vi "LVDT Thickness.vi"() -> ()   [LabVIEW 2014]
uses:
  <vilib>/Utility/miscctls.llb/LVBoundsTypeDef.ctl
  <vilib>/measure/NI_MABase.lvlib
panel:
  in  "stop":bool
  out "x >= y?":bool
  in  "Tab Control":T1(tab)
  out "Stage 2 Output":dbl(graph)
  out "Stage 1 Output":waveform(dbl)(graph)
  in  "?":bool
  in  "Slide":dbl(slide)=0.14061224489795918 scale=0.0..13.78
  out "?":dbl(slide) scale=0.0..15.0
  out "?":dbl format="%#_4g"
  out "?":dbl format="%#_4g"
  out "?":bool
  in  "?":bool
  out "?":dbl format="%#_4g"
  in  "?":dbl(slide)=29.292929292929294 scale=0.0..100.0
  out "?":dbl(slide) scale=0.0..15.0
  out "?":dbl format="%#_4g"
  out "Thickness (in mm) Vs Voltage (V)":cluster{"Y":dbl[], "Y":dbl[]}[](graph)
  out "1 2":string[][](table)
  out "?":bool
  out "Stage 1 Output  2":waveform(dbl)(graph)
  out "Stage 2 Output  2":dbl(graph)
  # "Manipal Institute of Technology  \n        Dept of Instrumentation and Control Engineering\n                                 V Sem (Instrumentation Lab)"
  # "VIRTUAL LABS"
  # "VIRTUAL LABS"
  # "Measurement of Level Using Ultrasonic Transducer\n \nAim:\nTo measure the liquid level in the process tank using Ultrasonic Transducer.\n Apparatus required:\n1\tVLMT-04 Unit.\n2\tPatch Chord.\n3\tDMM\n\n\nInstructions:\n1.\tSwitch ON the Trainer. \n2.\tThe Pump inlet valve (HV1) should be fully open and the process tank outlet valve HV2 should be fully closed. \n3.\tConnect the multimeter across (4-20) mA.\n4.\tVary the pump speed using variable speed knob, set the level at 0mm. \n5.\tNote the transmitter output in (4-20) mA terminals.\n6.\tGradually increase the water level by using variable speed knob and note down the water level and transmitter output.\n7.\tPlot the Graph between level (mm) and transmitter output (mA) along x-axis and y-axis respectively."
  # "EXPERIMENT NO.1"
  # "Thickness (mm)"
  # "Voltage o/p (V)"
  # "Thickness (mm)"
  # "Voltage o/p (V)"
  # "Animation Speed"
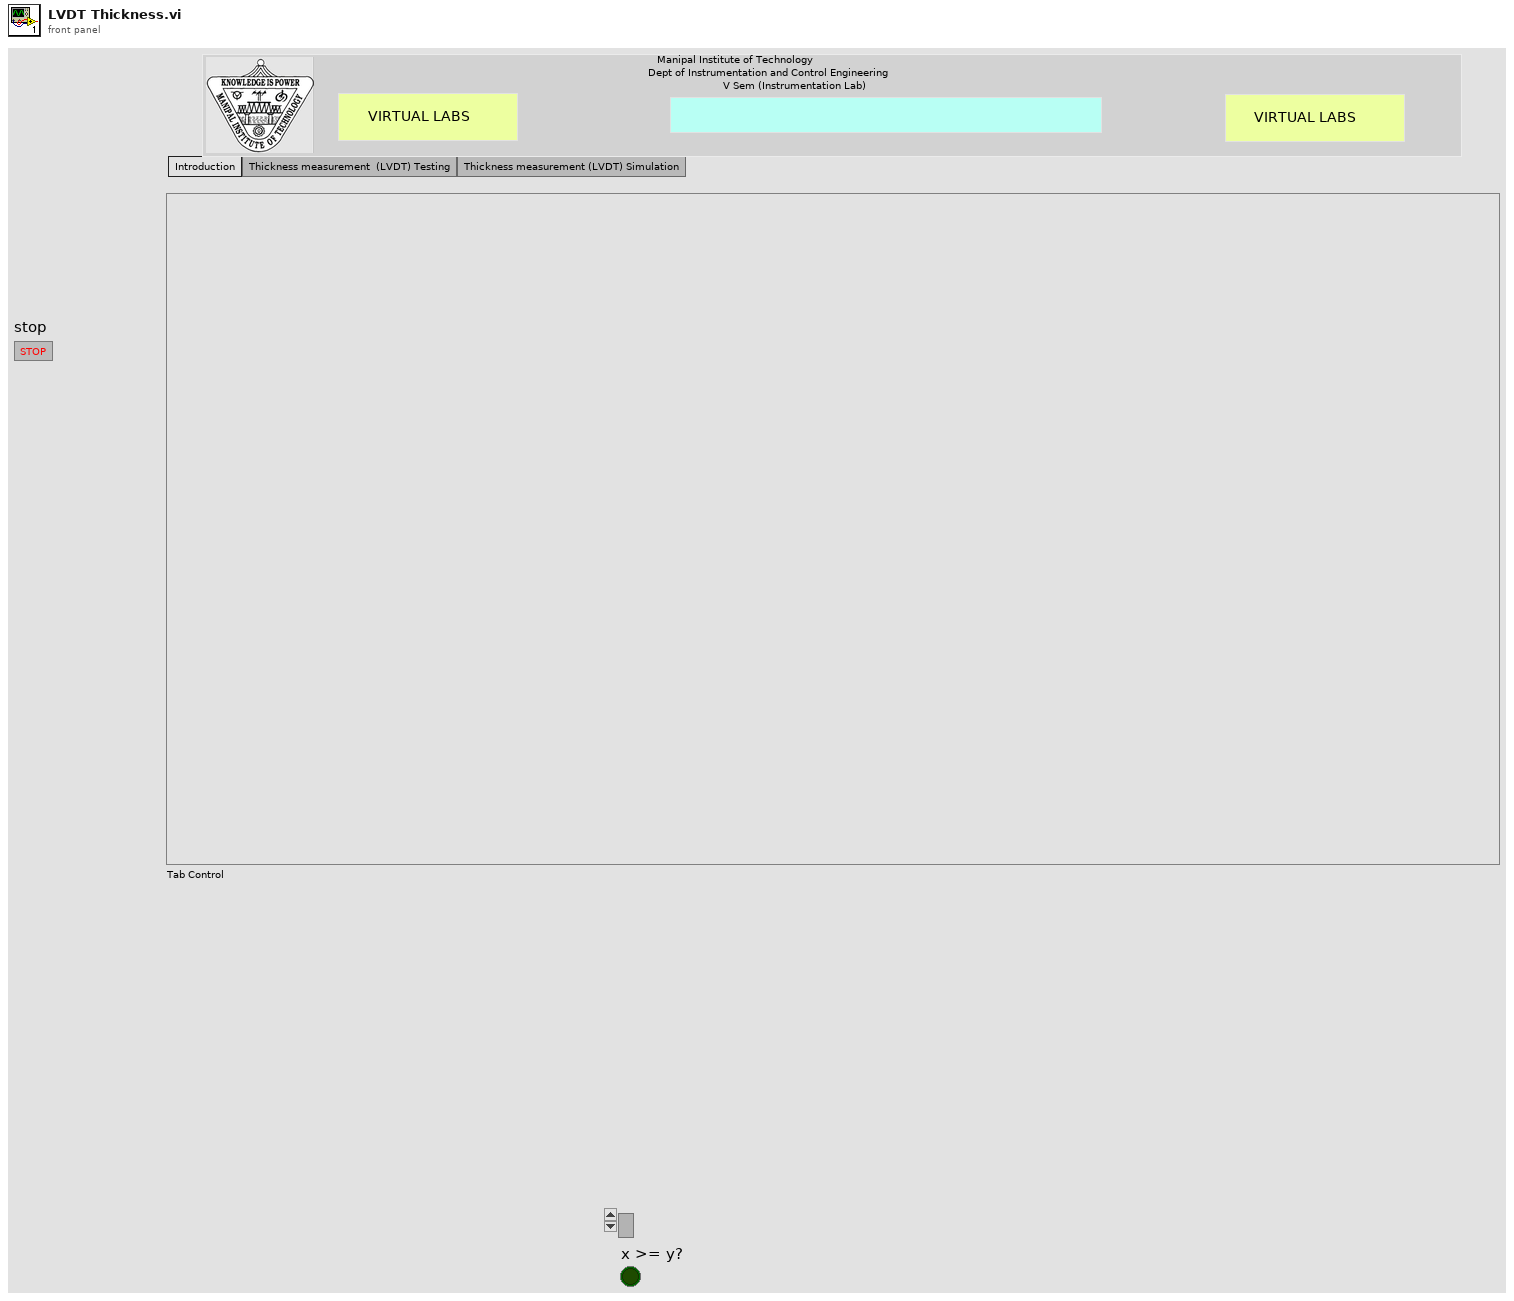
[diagram p1: front panel]
types:
  T1 = enum32{"Introduction", "Thickness measurement  (LVDT) Testing", "Thickness measurement (LVDT) Simulation"}
  T2 = typedef "LVBoundsTypeDef.ctl" = cluster{"Width":u32, "Height":u32}
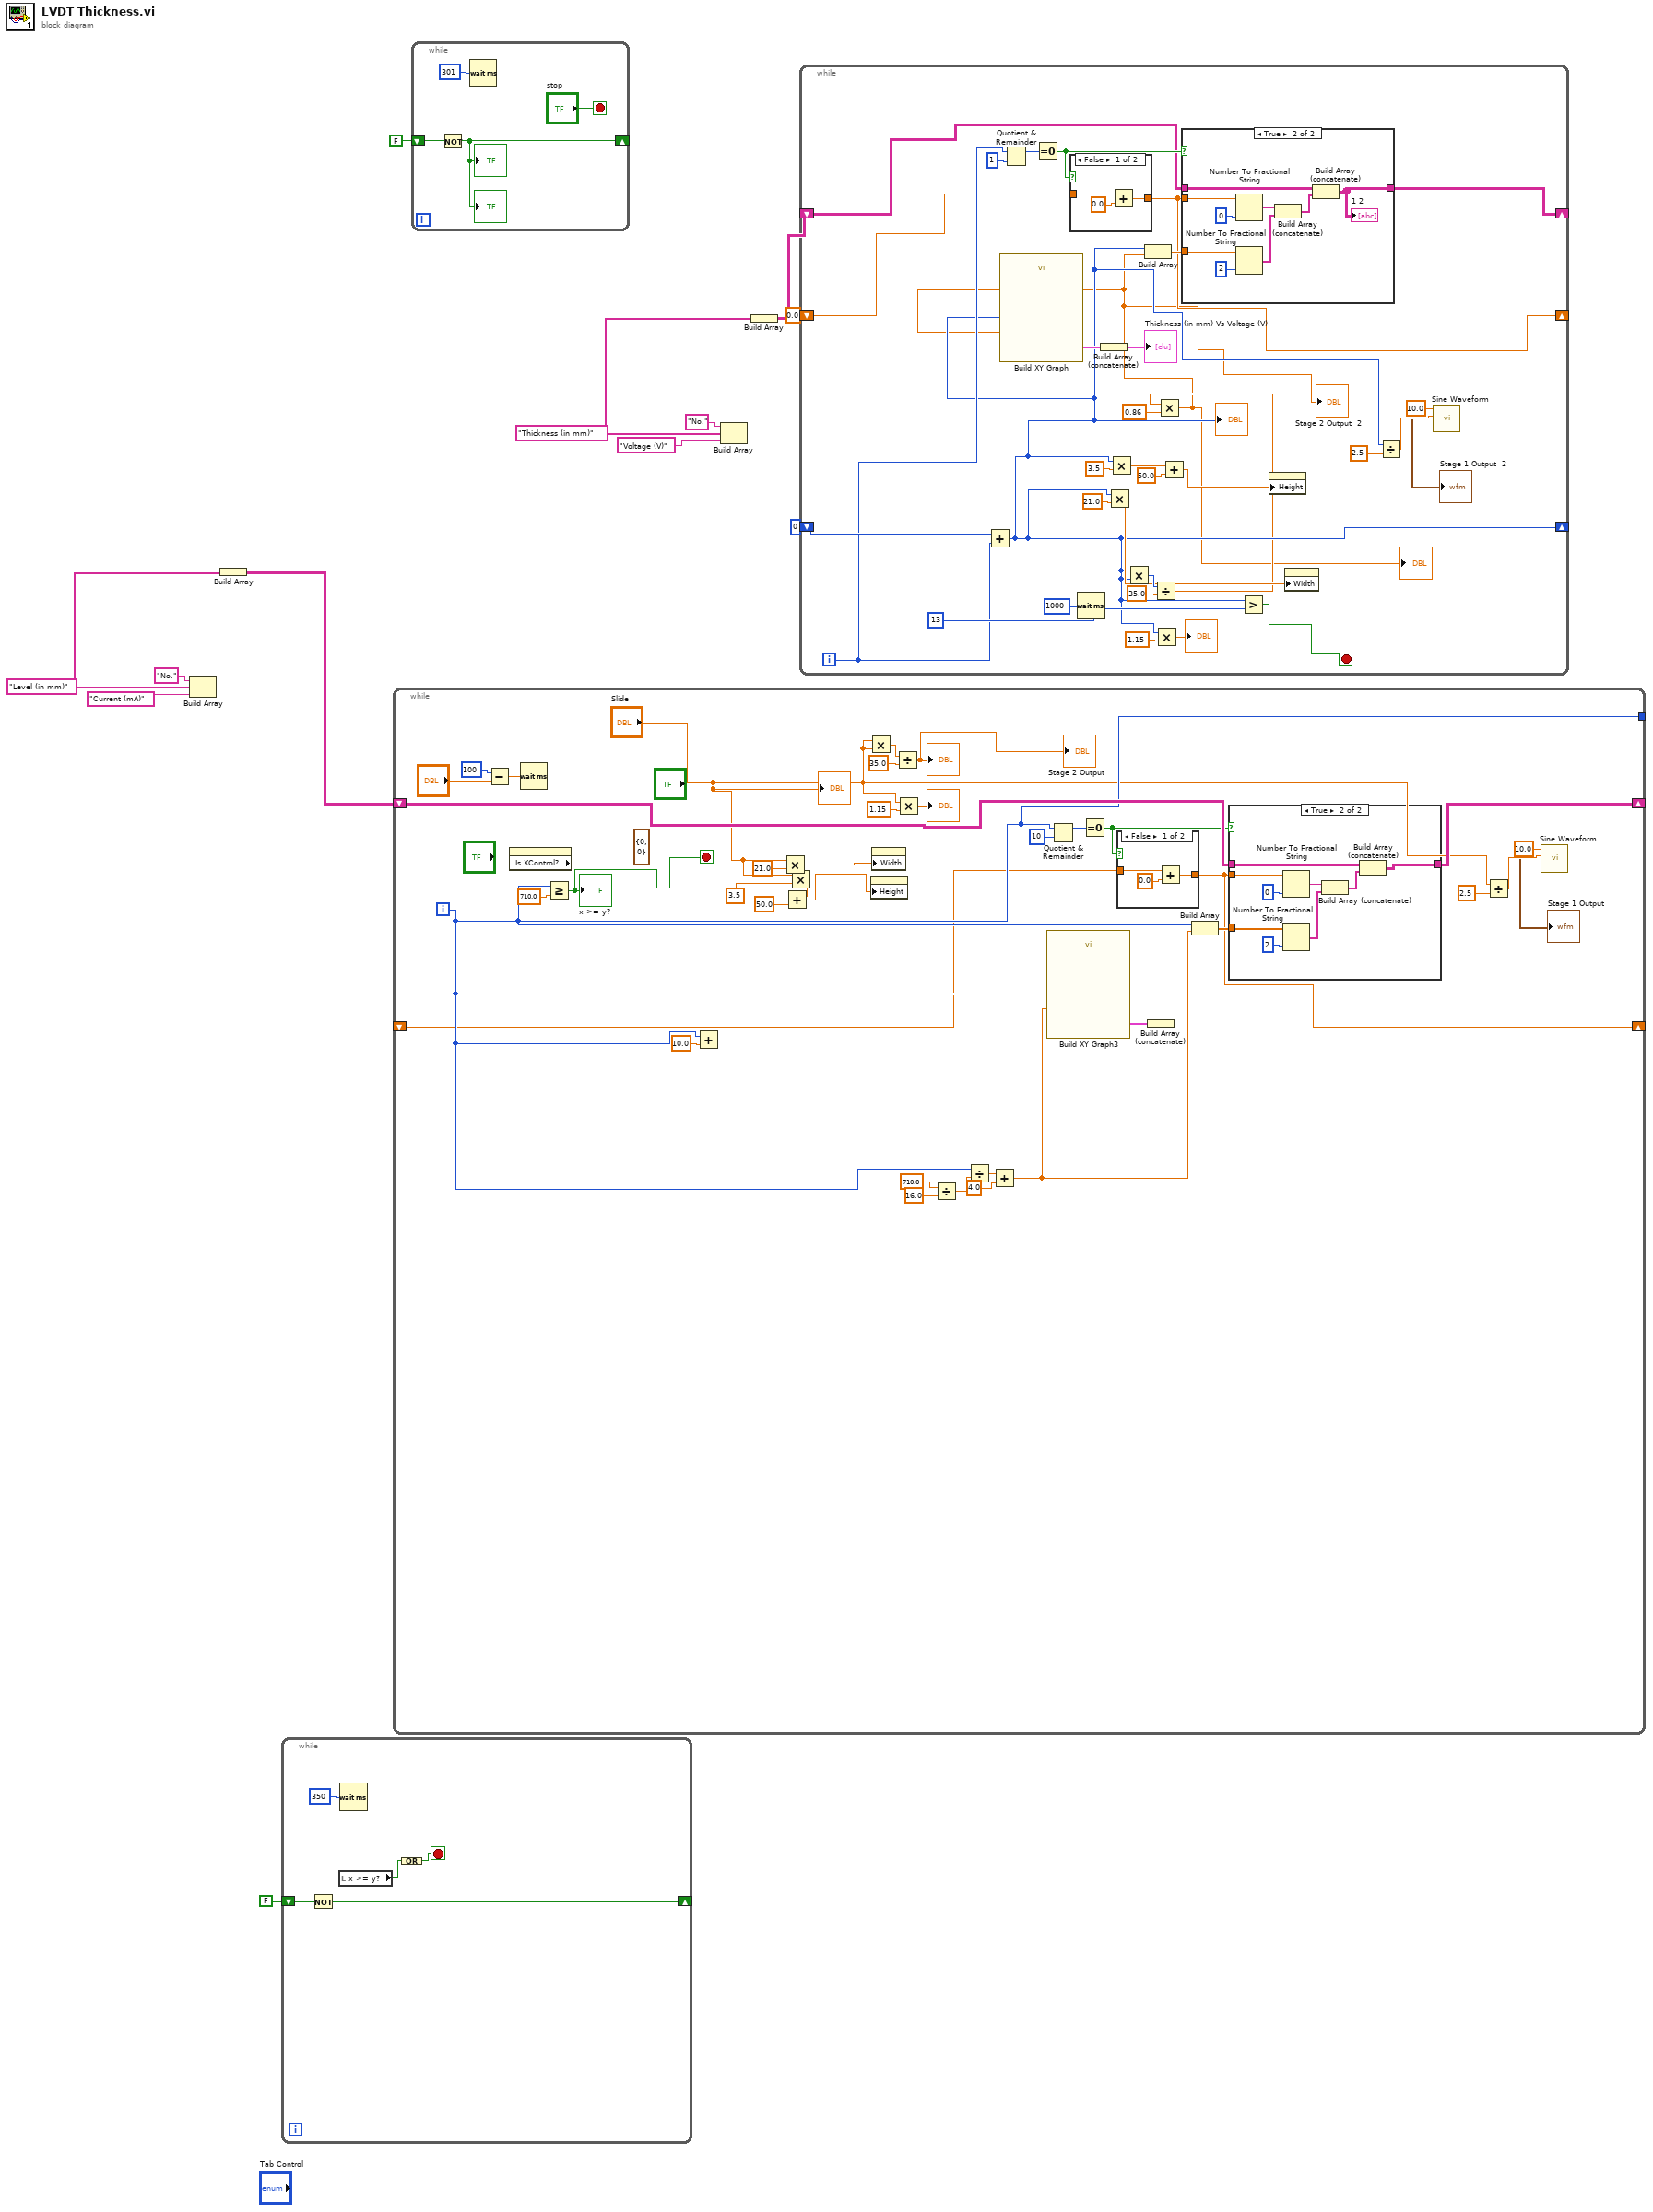
[diagram p0: block diagram]
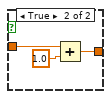
[diagram p2: hidden frame]
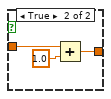
[diagram p4: hidden frame]
diagram:
  n1 = Build Array("No." ("element"), "Level (in mm)" ("element"), "Current (mA)") -> (w11:string[])
  n2 = Build Array(w11) -> (w10:string[][])
  n3 = while {
    shift-right: [w15] -> _
    shift-left: FALSE -> [w19]
    stop <- w16 stop-if-true
    n4 = Not(x=w19) -> (.not. x?=w15:bool)
    n5 = local read "x >= y?"() -> (w17:bool)
    n6 = Wait (ms)(milliseconds to wait=u32 350) -> ()  [unwired: 1 out]
    n7 = Compound Arithmetic op=OR(w17) -> (w16:bool)
  }
  n8 = while {
    tunnel: [w37] -> _
    shift-right: [w51] -> _
    shift-left: w10 -> [w52]
    shift-right: [w40] -> _
    shift-left: _ -> [w36]
    i -> [w37]
    stop <- w46 stop-if-true
    (unwired) T2 {"Width"=0, "Height"=0} ("XControl:Container Bounds")
    n9 = Subtract(x=u32 100 ("milliseconds to wait"), y="?") -> (x-y=w54:dbl)
    n10 = property class="Bool" props=["Is XControl?"]() -> ()  [unwired: 2 in, 3 out]
    n11 = Wait (ms)(milliseconds to wait=w54) -> ()  [unwired: 1 out]
    n12 = Greater Or Equal?(x=w37, y=710.0) -> (x >= y?=w46:bool)
    "x >= y?" <- w46
    n13 = Add(x=w37, y=10.0) -> ()  [unwired: 1 out]
    n14 = Multiply(x="Slide", y=21.0) -> (x*y=w33:dbl)
    n15 = Multiply(x="Slide", y=3.5) -> (x*y=w32:dbl)
    n16 = Add(x=w32, y=50.0) -> (x+y=w31:dbl)
    n17 = Multiply(x="Slide", y="Slide") -> (x*y=w27:dbl)
    n18 = property class="Bool"("Height"=w31) -> ()  [unwired: 2 in, 2 out]
    n19 = property class="Bool"("Width"=w33) -> ()  [unwired: 2 in, 2 out]
    n20 = Divide(x=w27, y=35.0 ("x*y")) -> (x/y=→"?" →"Stage 2 Output":dbl)
    n21 = Multiply(x="Slide", y=1.15) -> (x*y=→"?":dbl)
    n22 = Divide(x=710.0, y=16.0) -> (x/y=w43:dbl)
    n23 = Divide(x=w37, y=w43) -> (x/y=w42:dbl)
    n24 = Add(x=w42, y=4.0) -> (x+y=w38:dbl)
    n25 = call "Build XY Graph3"("Y Input"=w38, "X Input"=w37) -> ("XY Graph"=w56:cluster{"Y":dbl[], "Y":dbl[]}[])  [unwired: 3 in, 6 out]
    n26 = Quotient & Remainder(x=w37, y=10) -> (x-y*floor(x/y)=w50:i32)  [unwired: 1 out]
    n27 = Equal To 0?(x=w50) -> (x = 0?=w47:bool)
    n28 = case shown="False" w47 {
      tunnel: w36 -> [w59 w63]
      tunnel: [w58 w62] -> w40
      frame False {
        n29 = Add(x=w59, y=0.0) -> (x+y=w58:dbl)
      }
      frame True {
        n30 = Add(x=w63, y=1.0) -> (x+y=w62:dbl)
      }
    }
    n31 = Build Array (concatenate)(w56) -> ()  [unwired: 1 out]
    n32 = Build Array(w37, w38) -> (w48:dbl[])
    n33 = case shown="True" w47 {
      tunnel: w48 -> [_ w73]
      tunnel: w52 -> [w64 w66]
      tunnel: [w64 w65] -> w51
      tunnel: w40 -> [_ w71]
      frame False {
      }
      frame True {
        n34 = Number To Fractional String(number=w71, precision (6)=i16 0) -> (F-format string=w69:string)  [unwired: 2 in]
        n35 = Number To Fractional String(number=w73, precision (6)=i16 2) -> (F-format string=w68:string[])  [unwired: 2 in]
        n36 = Build Array (concatenate)(w69, w68) -> (w67:string[])
        n37 = Build Array (concatenate)(w66, w67) -> (w65:string[][])
      }
    }
    n38 = Divide(x="Slide", y=2.5) -> (x/y=w23:dbl)
    n39 = call <vilib>:"Sine Waveform.vi"("amplitude"=w23, "frequency"=10.0) -> ("signal out"=→"Stage 1 Output":waveform(dbl))  [unwired: 8 in, 1 out]
    "?" <- "Slide"
  }
  n40 = while {
    shift-right: [w75] -> _
    shift-left: FALSE -> [w77]
    stop <- "stop" stop-if-true
    n41 = Not(x=w77) -> (.not. x?=w75:bool)
    "?" <- w75
    "?" <- w75
    n42 = Wait (ms)(milliseconds to wait=u32 301) -> ()  [unwired: 1 out]
  }
  n43 = Build Array("No." ("element"), "Thickness (in mm)" ("element"), "Voltage (V)") -> (w7:string[])
  n44 = Build Array(w7) -> (w4:string[][])
  n45 = while {
    shift-right: [w80] -> _
    shift-left: 0 -> [w110]
    shift-right: [w86] -> _
    shift-left: w4 -> [w90]
    shift-right: [w89] -> _
    shift-left: 0.0 -> [w87]
    i -> [w88]
    stop <- w97 stop-if-true
    n46 = Add(x=w110, y=w88) -> (x+y=w80:i32)
    "?" <- w80
    n47 = Quotient & Remainder(x=w88, y=1) -> (x-y*floor(x/y)=w95:i32)  [unwired: 1 out]
    n48 = Equal To 0?(x=w95) -> (x = 0?=w92:bool)
    n49 = case shown="False" w92 {
      tunnel: [w112 w116] -> w89
      tunnel: w87 -> [w111 w114]
      frame False {
        n50 = Add(x=w111, y=0.0) -> (x+y=w112:dbl)
      }
      frame True {
        n51 = Add(x=w114, y=1.0) -> (x+y=w116:dbl)
      }
    }
    n52 = Wait (ms)(milliseconds to wait=u32 1000) -> ()  [unwired: 1 out]
    n53 = Multiply(x=w80, y=21.0) -> (x*y=w99:dbl)
    n54 = Multiply(x=w80, y=3.5) -> (x*y=w103:dbl)
    n55 = Multiply(x=w80, y=w80) -> (x*y=w108:i32)
    n56 = Divide(x=w108, y=35.0 ("x*y")) -> (x/y=w79:dbl)
    n57 = Multiply(x=w80, y=1.15) -> (x*y=→"?":dbl)
    n58 = Multiply(x=w79, y=0.86) -> (x*y=w78:dbl)
    "?" <- w78
    "Stage 2 Output  2" <- w78
    n59 = call "Build XY Graph"("Y Input"=w78, "X Input"=w80) -> ("XY Graph"=w96:cluster{"Y":dbl[], "Y":dbl[]}[])  [unwired: 3 in, 6 out]
    n60 = Build Array (concatenate)(w96) -> (→"Thickness (in mm) Vs Voltage (V)":cluster{"Y":dbl[], "Y":dbl[]}[])
    n61 = Build Array(w80, w78) -> (w93:dbl[])
    n62 = Add(x=w103, y=50.0) -> (x+y=w100:dbl)
    n63 = case shown="True" w92 {
      tunnel: w93 -> [_ w118]
      tunnel: w90 -> [w117 w120]
      tunnel: [w117 w119] -> w86
      tunnel: w89 -> [_ w125]
      frame False {
      }
      frame True {
        n64 = Number To Fractional String(number=w125, precision (6)=i16 0) -> (F-format string=w123:string)  [unwired: 2 in]
        n65 = Number To Fractional String(number=w118, precision (6)=i16 2) -> (F-format string=w122:string[])  [unwired: 2 in]
        n66 = Build Array (concatenate)(w123, w122) -> (w121:string[])
        n67 = Build Array (concatenate)(w120, w121) -> (w119:string[][])
        "1 2" <- w119
      }
    }
    n68 = Greater?(x=w80, y=13) -> (0:w97:bool)
    n69 = property class="Bool"("Height"=w100) -> ()  [unwired: 2 in, 2 out]
    n70 = property class="Bool"("Width"=w99) -> ()  [unwired: 2 in, 2 out]
    n71 = Divide(x=w80, y=2.5) -> (x/y=w83:dbl)
    n72 = call <vilib>:"Sine Waveform.vi"("amplitude"=w83, "frequency"=10.0) -> ("signal out"=→"Stage 1 Output  2":waveform(dbl))  [unwired: 8 in, 1 out]
  }
